vi "AO.vi"() -> ()   [LabVIEW 2012]
uses:
  <vilib>/Utility/error.llb/DialogType.ctl
  <vilib>/DAQmx/write.llb/DAQmx Write (Analog 1D Wfm NChan NSamp).vi
  <vilib>/DAQmx/create/channels.llb/DAQmx Create Channel (AO-Voltage-Basic).vi
  <vilib>/DAQmx/configure/timing.llb/DAQmx Timing (Sample Clock).vi
  <vilib>/DAQmx/configure/trigger.llb/DAQmx Start Trigger (Digital Edge).vi
  <vilib>/DAQmx/configure/trigger.llb/DAQmx Start Trigger (Analog Edge).vi
  <vilib>/DAQmx/miscellaneous.llb/DAQmx Fill In Error Info.vi
  <resource>/objmgr/daqmx.rc
panel:
  out "x-y":dbl
  in  "Offset":dbl=4.975
  out "Waveform Graph 2":dynamicdata(graph)
  in  "Trigger Type 2":T1(tab)
  in  "Edge 2":i32(ring)=10280 items=["Rising"=10280, "Falling"=10171]
  in  "Digital Trigger Source 2":tag
  in  "Level (V) 2":dbl format="%0.2f"
  in  "Hysteresis (V) 2":dbl
  in  "Slope 2":i32(ring)=10280 items=["Rising"=10280, "Falling"=10171]
  in  "Analog Trigger Source 2":string="APFI0"
  in  "Pause When":i32(ring)=10192 items=["High"=10192, "Low"=10214]
  in  "Pause Trigger Source":tag
  in  "Sample Rate 2":dbl=1000.0
  in  "Sample Clock Source 2":tag="OnboardClock"
  in  "Max Voltage 2":dbl=5.0
  in  "Min Voltage 2":dbl=-5.0
  in  "Physical Channel(s)":tag="Dev1/ao0"
  out "Actual Sample Rate 2":dbl=1000.0 format="%0.2f"
  # "To configure and use a start trigger you must have the necessary tab selected above.  Not all hardware supports triggering--refer to your device documentation for more info."
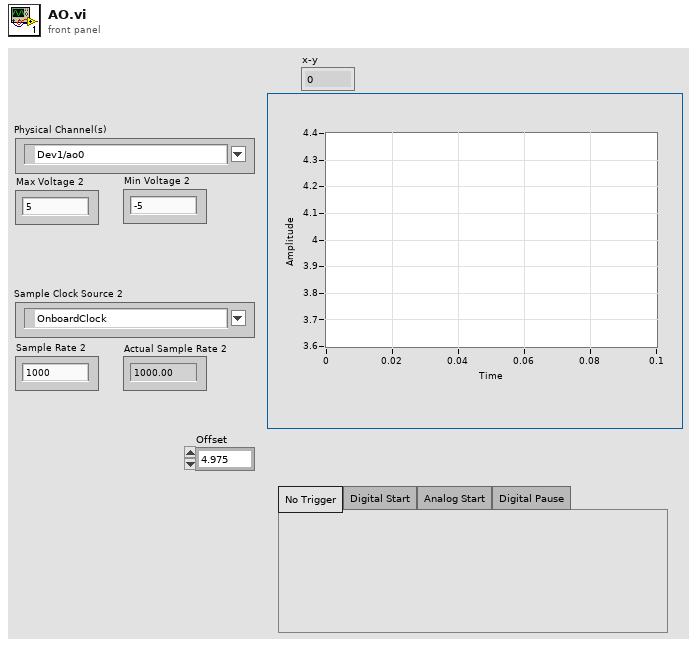
[diagram p1: front panel]
types:
  T1 = enum32{"No Trigger", "Digital Start", "Analog Start", "Digital Pause"}
  T2 = typedef "DialogType.ctl" = u16
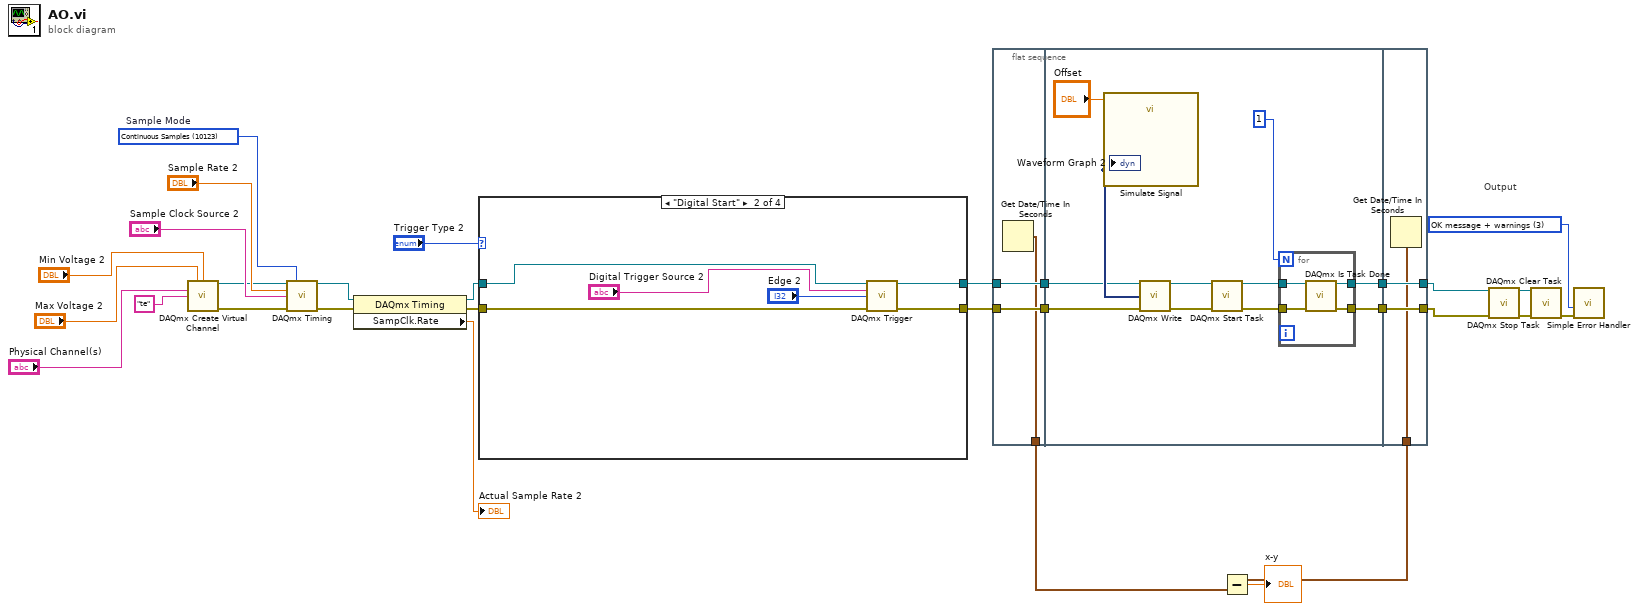
[diagram p0: block diagram]
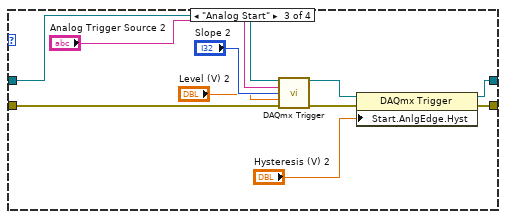
[diagram p3: hidden frame]
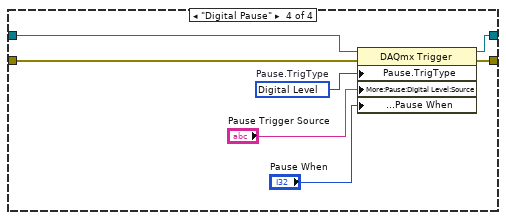
[diagram p4: hidden frame]
diagram:
  w29 = T2 3 items=["no dialog", "OK message", "continue or stop message", "OK message + warnings", "continue/stop + warnings"] ("type of dialog (OK msg:1)")
  w13 = 10123 items=["Finite Samples"=10178, "Continuous Samples"=10123, "Hardware Timed Single Point"=12522]  # Sample Mode
  # "Output"
  n1 = call-poly <vilib>:"DAQmx Create Virtual Channel.vi"("maximum value"="Max Voltage 2", "minimum value"="Min Voltage 2", "physical channels"="Physical Channel(s)", "name to assign"="te") -> ("task out"=w15:refnum<k21>, "error out"=w14:errorcluster)  [unwired: 10 in]
  n2 = call-poly <vilib>:"DAQmx Timing.vi"("task/channels in"=w15, "sample mode"=w13, "rate"="Sample Rate 2", "source"="Sample Clock Source 2", "error in"=w14) -> ("task out"=w11:refnum<k21>, "error out"=w12:errorcluster)  [unwired: 9 in]
  n3 = property class="DAQmx Timing"(reference=w11, error in=w12) -> (reference out=w23:refnum<k21>, error out=w24:errorcluster, "SampClk.Rate"=→"Actual Sample Rate 2":dbl)
  n4 = case shown="\"Digital Start\"" "Trigger Type 2" {
    tunnel: w23 -> [w32 w38 w48 w55]
    tunnel: w24 -> [w31 w37 w47 w52]
    tunnel: [w32 w36 w45 w54] -> w26
    tunnel: [w31 w35 w44 w53] -> w30
    frame "No Trigger", Default {
    }
    frame "Digital Start" {
      n5 = call-poly <vilib>:"DAQmx Trigger.vi"("task/channels in"=w38, "source"="Digital Trigger Source 2", "edge"="Edge 2", "error in"=w37) -> ("task out"=w36:refnum<k21>, "error out"=w35:errorcluster)  [unwired: 10 in]
    }
    frame "Analog Start" {
      n6 = call-poly <vilib>:"DAQmx Trigger.vi"("task/channels in"=w48, "source"="Analog Trigger Source 2", "slope"="Slope 2", "level"="Level (V) 2", "error in"=w47) -> ("task out"=w43:refnum<k21>, "error out"=w42:errorcluster)  [unwired: 9 in]
      n7 = property class="DAQmx Trigger"(reference=w43, error in=w42, "Start.AnlgEdge.Hyst"="Hysteresis (V) 2") -> (reference out=w45:refnum<k21>, error out=w44:errorcluster)
    }
    frame "Digital Pause" {
      w51 = 10152 items=["Analog Level"=10101, "Analog Window"=10103, "Digital Level"=10152, "Digital Pattern"=10398, "None"=10230]  # Pause.TrigType
      n8 = property class="DAQmx Trigger"(reference=w55, error in=w52, "Pause.TrigType"=w51, "More:Pause:Digital Level:Source"="Pause Trigger Source", "More:Pause:Digital Level:Pause When"="Pause When") -> (reference out=w54:refnum<k21>, error out=w53:errorcluster)
    }
  }
  n9 = flat-sequence {
    tunnel: w26 -> [w57]
    tunnel: w30 -> [w58]
    tunnel: [w58] -> w7
    tunnel: [w57] -> w6
    tunnel: [w56] -> w2
    tunnel: w7 -> [w69]
    tunnel: w6 -> [w65]
    tunnel: [w62] -> w5
    tunnel: [w60] -> w4
    tunnel: [w75] -> w8
    tunnel: [w76] -> w9
    tunnel: w5 -> [w76]
    tunnel: w4 -> [w75]
    tunnel: [w74] -> w3
    frame #0 {
      n10 = Get Date/Time In Seconds() -> (seconds since 1Jan1904=w56:timestamp)
    }
    frame #1 {
      n11 = call "Simulate Signal"("Offset"="Offset") -> ("DC"=w68:dynamicdata)  [unwired: 13 in, 1 out]
      "Waveform Graph 2" <- w68
      n12 = call-poly <vilib>:"DAQmx Write.vi"("task/channels in"=w65, "data"=w68, "error in"=w69) -> ("task out"=w66:refnum<k21>, "error out"=w67:errorcluster)  [unwired: 10 in, 1 out]
      n13 = call <vilib>:"DAQmx Start Task.vi"("task/channels in"=w66, "error in"=w67) -> ("task out"=w63:refnum<k21>, "error out"=w61:errorcluster)  [unwired: 12 in]
      n14 = for {
        N: 1 -> [_]
        tunnel: w63 -> [w73]
        tunnel: [w72] -> w62
        tunnel: w61 -> [w71]
        tunnel: [w70] -> w60
        n15 = call <vilib>:"DAQmx Is Task Done.vi"("task/channels in"=w73, "error in"=w71) -> ("task out"=w72:refnum<k21>, "error out"=w70:errorcluster)  [unwired: 11 in, 1 out]
      }
    }
    frame #2 {
      n16 = Get Date/Time In Seconds() -> (seconds since 1Jan1904=w74:timestamp)
    }
  }
  n17 = Subtract(x=w3, y=w2) -> (x-y=→"x-y":dbl)
  n18 = call <vilib>:"DAQmx Stop Task.vi"("task/channels in"=w9, "error in"=w8) -> ("task out"=w27:refnum<k21>, "error out"=w28:errorcluster)  [unwired: 12 in]
  n19 = call <vilib>:"DAQmx Clear Task.vi"("task in"=w27, "error in"=w28) -> ("error out"=w16:errorcluster)  [unwired: 13 in]
  n20 = call <vilib>:"Simple Error Handler.vi"("type of dialog (OK msg:1)"=w29, "error in (no error)"=w16) -> ()  [unwired: 3 in, 5 out]
